vi "Commit Tool Config.vi"(8 "error in (no error)":errorcluster, 9 "Tool Config Cluster":T1={"Tool Type"=0, "Tool SN"=0, "Tool Block"={"Encoder Size"=0, "Encoder Scale"=0, "Encoder Offset"=0, "MaxEncoder"=0, "MinEncoder"=0, "Start Delay"=0.0, "Tool Face Ref"=0.0}, "Motor Block"={"MinMotor Speed"=0, "MaxMotor Speed"=0, "Homing Speed"=90, "Jog Speed"=90, "Inspect Speed"=90, "VBlk Speed"=90, "CleaningPos"=0, "Safe Zone"=0, "Has Motor"=FALSE, "Use Home Index"=FALSE}, "Verification Block"={"Angle"=90.0, "FlankLength1"=0.0, "FlankLength2"=0.0, "Location"=0.0, "Serial Number"=0}, "Probe Block"={"nProbes"=0, "Probe Param Array"=[]}} {"Probe Block"."Probe Param Array"."Sensor Block"."SensorCfgParams Array"."CalibrCoefArray" format="%#.12g"}) -> (0 "error out":errorcluster)   [LabVIEW 2015, in "Tool Module.lvlib"]
doc: "<b>Note</b>: This VI was renamed by the DQMH Rename Event utility. Make sure the VI Description is updated to reflect the new event name, then delete this comment.\n\nSaves Tool Configuration to Tool. If Commit is True it stores to File system, otherwise just update memory copy.\n_____\nCreated using Delacor QMH Event Scripter 3.1.0.29."
uses:
  Tool Module.lvlib
  Tool Config/_Configuration Cluster_v3--typedef.ctl
  Tool Config/_Tool Block Cluster_v3--typedef.ctl
  Tool Config/_Motor Block Cluster_v2--typedef.ctl
  Tool Config/_Verification Blk Cluster--typedef.ctl
  Tool Config/_ProbeConfigParams Cluster--typedef.ctl
  Tool Config/_Sensor Block Cluster--typedef.ctl
  Tool Config/_SensorConfigParams Cluster--typedef.ctl
  Commit Tool Config Argument--cluster.ctl
  Tool Config/Tool Cfg.lvlib
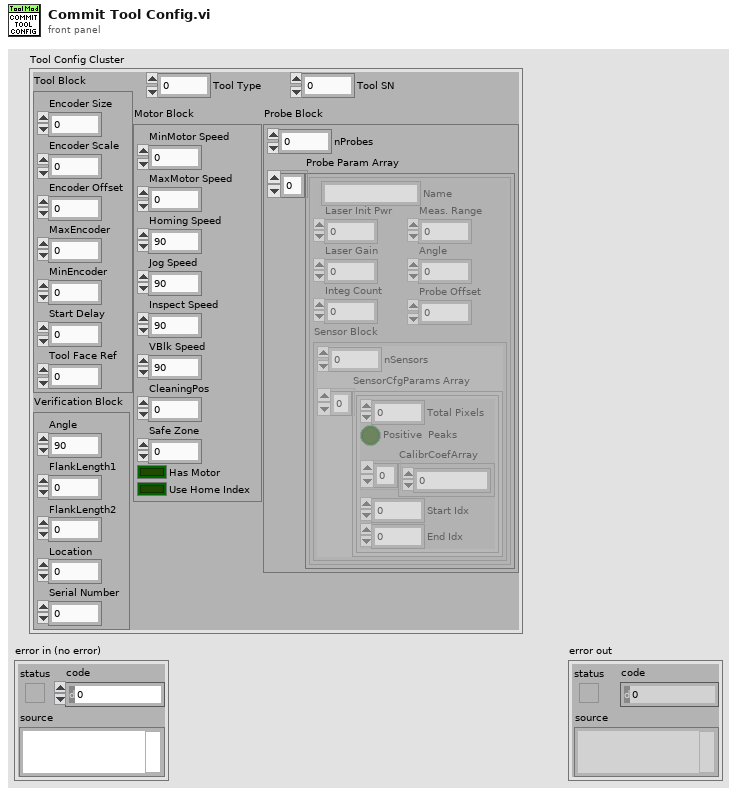
[diagram p1: front panel]
types:
  T1 = typedef "Tool Cfg.lvlib/_Configuration Cluster_v3--typedef.ctl" = cluster{"Tool Type":u16, "Tool SN":u16, "Tool Block":T2, "Motor Block":T3, "Verification Block":T4, "Probe Block":cluster{"nProbes":u16, "Probe Param Array":T5[]}}
  T2 = typedef "Tool Cfg.lvlib/_Tool Block Cluster_v3--typedef.ctl" = cluster{"Encoder Size":u16, "Encoder Scale":u32, "Encoder Offset":i32, "MaxEncoder":i32, "MinEncoder":i32, "Start Delay":sgl, "Tool Face Ref":sgl}
  T3 = typedef "Tool Cfg.lvlib/_Motor Block Cluster_v2--typedef.ctl" = cluster{"MinMotor Speed":u16, "MaxMotor Speed":u16, "Homing Speed":u16, "Jog Speed":u16, "Inspect Speed":u16, "VBlk Speed":u16, "CleaningPos":i32, "Safe Zone":i32, "Has Motor":bool, "Use Home Index":bool}
  T4 = typedef "Tool Cfg.lvlib/_Verification Blk Cluster--typedef.ctl" = cluster{"Angle":sgl, "FlankLength1":sgl, "FlankLength2":sgl, "Location":sgl, "Serial Number":u16}
  T5 = typedef "Tool Cfg.lvlib/_ProbeConfigParams Cluster--typedef.ctl" = cluster{"Name":string, "Laser Init Pwr":u16, "Laser Gain":u8, "Integ Count":u16, "Meas. Range":sgl, "Angle":sgl, "Probe Offset":sgl, "Sensor Block":T6}
  T6 = typedef "Tool Cfg.lvlib/_Sensor Block Cluster--typedef.ctl" = cluster{"nSensors":u16, "SensorCfgParams Array":T7[]}
  T7 = typedef "Tool Cfg.lvlib/_SensorConfigParams Cluster--typedef.ctl" = cluster{"Total Pixels":u16, "Positive  Peaks":bool, "CalibrCoefArray":dbl[], "Start Idx":u16, "End Idx":u16}
  T8 = typedef "Tool Module.lvlib/Commit Tool Config Argument--cluster.ctl" = cluster{"Tool Config Cluster":T1}
  T9 = typedef "Tool Module.lvlib/Request Events--cluster.ctl" = cluster{"Stop Module":refnum<user-event>, "Show Panel":refnum<user-event>, "Hide Panel":refnum<user-event>, "Get Module Execution Status":refnum<user-event>, "Show Diagram":refnum<user-event>, "GOTO":refnum<user-event>, "CONNECT":refnum<user-event>, "Get All Inspect Data":refnum<user-event>, "Start Data Monitor":refnum<user-event>, "Get FPGA Setup Params":refnum<user-event>, "Set FPGA Setup Params":refnum<user-event>, "Commit Tool Config":refnum<user-event>, "Set Integration Count":refnum<user-event>, "Set Laser Params":refnum<user-event>, "Get Mtrl Ctrl Reg":refnum<user-event>, "Commit Ctrl Reg":refnum<user-event>, "Set Event Logger":refnum<user-event>, "Write to File":refnum<user-event>, "Read from File":refnum<user-event>, "Set Device Temp Thresholds":refnum<user-event>, "Get Cycle Count":refnum<user-event>, "Return FPGA Setup Data":refnum<user-event>, "Update FPGA Setup Data":refnum<user-event>, "Setup Timer":refnum<user-event>, "Tool Status Reader Cmd":refnum<user-event>, "Stop Helper Loops":refnum<user-event>, "Enable Receive Stream":refnum<user-event>, "Get-Set Inspection Limits":refnum<user-event>, "INSPECT":refnum<user-event>}
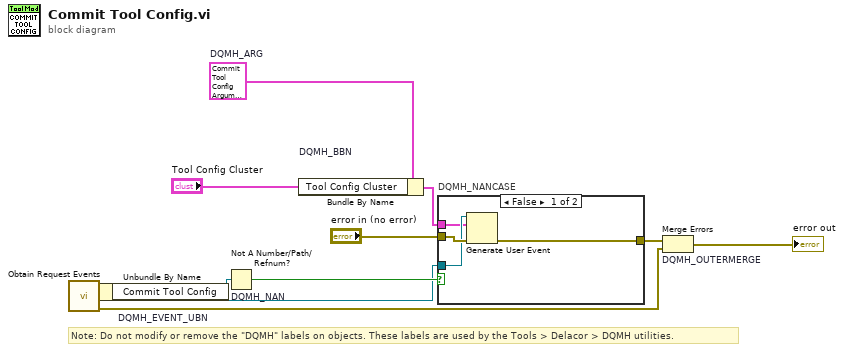
[diagram p0: block diagram]
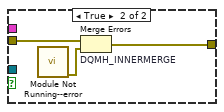
[diagram p2: hidden frame]
diagram:
  w4 = T8 {"Tool Config Cluster"={"Tool Type"=0, "Tool SN"=0, "Tool Block"={"Encoder Size"=0, "Encoder Scale"=0, "Encoder Offset"=0, "MaxEncoder"=0, "MinEncoder"=0, "Start Delay"=0.0, "Tool Face Ref"=0.0}, "Motor Block"={"MinMotor Speed"=0, "MaxMotor Speed"=0, "Homing Speed"=90, "Jog Speed"=90, "Inspect Speed"=90, "VBlk Speed"=90, "CleaningPos"=0, "Safe Zone"=0, "Has Motor"=FALSE, "Use Home Index"=FALSE}, "Verification Block"={"Angle"=90.0, "FlankLength1"=0.0, "FlankLength2"=0.0, "Location"=0.0, "Serial Number"=0}, "Probe Block"={"nProbes"=0, "Probe Param Array"=[]}}}  # DQMH_ARG
  # "Note: Do not modify or remove the \"DQMH\" labels on objects. These labels are used by the Tools > Delacor > DQMH utilities."
  n1 = call "Obtain Request Events.vi"() -> ("error out"=w2:errorcluster, "Tool Module Request Events"=w1:T9)  [unwired: 10 in]
  n2 = Unbundle By Name "DQMH_EVENT_UBN"(w1) -> ("Commit Tool Config"=w6:refnum<user-event>)
  n3 = Not A Number/Path/Refnum? "DQMH_NAN"(number/path/refnum=w6) -> (NaN/Path/Refnum?=w7:bool)
  n4 = Bundle By Name "DQMH_BBN"(cluster=w4, "Tool Config Cluster"="Tool Config Cluster") -> (w8:T8)
  n5 = case "DQMH_NANCASE" shown="False" w7 {
    tunnel: "error in (no error)" -> [w14 w17]
    tunnel: [w13 w16] -> w5
    tunnel: w6 -> [w12 _]
    tunnel: w8 -> [w11 _]
    frame False {
      n6 = Generate User Event(user event=w12, event data cluster=w11, error in=w14) -> (error out=w13:errorcluster)  [unwired: 1 in, 1 out]
    }
    frame True {
      n7 = call "Module Not Running--error.vi"() -> ("error out"=w15:errorcluster)  [unwired: 11 in]
      n8 = Merge Errors "DQMH_INNERMERGE"(w17, w15) -> (w16:errorcluster)
    }
  }
  n9 = Merge Errors "DQMH_OUTERMERGE"(w5, w2) -> (→"error out":errorcluster)
